vi "Init ConvBox Handler.vi"(8 "error in (no error)":errorcluster, 11 "Listener in":refnum<class "Listener.lvclass">) -> (0 "error out":errorcluster, 3 "Listener out":refnum<class "Listener.lvclass">)   [LabVIEW 2023, in "Listener.lvclass"]
uses:
  Listener.lvclass
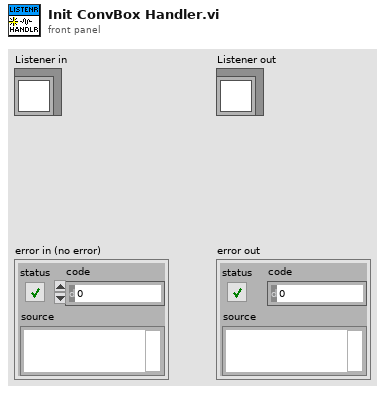
[diagram p1: front panel]
types:
  T1 = typedef "Listener.lvclass/RS-xxx To GPIB ConvBox Data Structure.ctl" = cluster{"Data":string, "Command Messages Read":string[], "Address":string, "Data Length":u32}
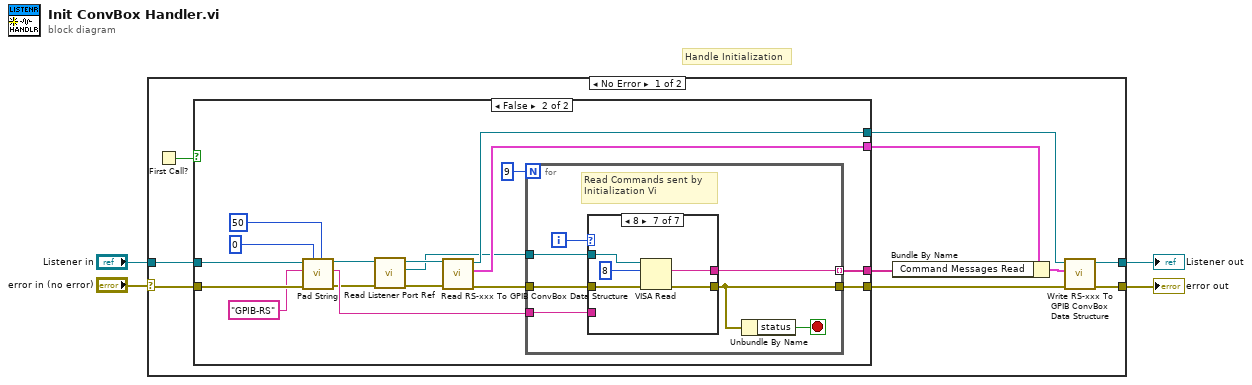
[diagram p0: block diagram]
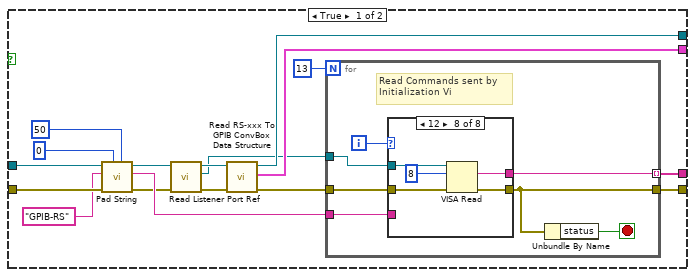
[diagram p2: hidden frame]
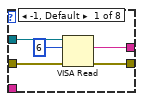
[diagram p3: hidden frame]
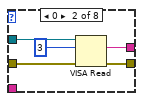
[diagram p4: hidden frame]
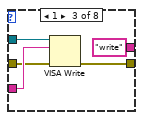
[diagram p5: hidden frame]
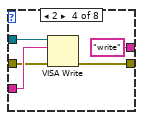
[diagram p6: hidden frame]
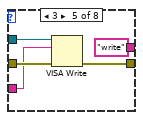
[diagram p7: hidden frame]
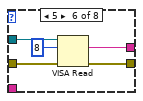
[diagram p8: hidden frame]
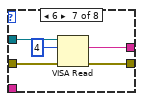
[diagram p9: hidden frame]
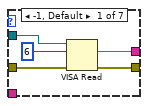
[diagram p10: hidden frame]
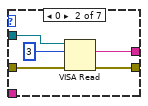
[diagram p11: hidden frame]
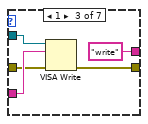
[diagram p12: hidden frame]
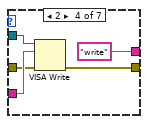
[diagram p13: hidden frame]
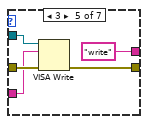
[diagram p14: hidden frame]
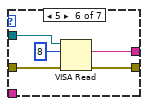
[diagram p15: hidden frame]
diagram:
  # "Handle Initialization"
  n1 = case shown="No Error" "error in (no error)" {
    selector: "error in (no error)" -> [w14 w139]
    tunnel: [w5 w139] -> w4
    tunnel: "Listener in" -> [w12 w138]
    tunnel: [w10 w138] -> w1
    frame No Error {
      n2 = First Call?() -> (First Call?: T/F=w13:bool)
      n3 = case shown="False" w13 {
        tunnel: [w31 w95] -> w6
        tunnel: w14 -> [w27 w91]
        tunnel: w12 -> [w22 w90]
        tunnel: [w29 w93] -> w11
        tunnel: [w21 w84] -> w9
        tunnel: [w20 w85] -> w8
        frame True {
          n4 = call "Pad String.vi"("Expected Length"=u8 50 ("Pad Character"), "Pad Character"=u8 0 ("Expected Length"), "error in (no error)"=w27, "String To Pad"="GPIB-RS" ("search string/char (-)"), "Listener in"=w22) -> ("error out"=w19:errorcluster, "Padded String"=w23:string, "Listener out"=w17:refnum<class "Listener.lvclass">)  [unwired: 4 in]
          n5 = call "Read Listener Port Ref.vi"("error in (no error)"=w19, "Listener in"=w17) -> ("error out"=w18:errorcluster, "Listener Port Ref"=w15:refnum<visa-resource-name>, "Listener out"=w16:refnum<class "Listener.lvclass">)  [unwired: 7 in]
          n6 = call-dynamic "Read RS-xxx To GPIB ConvBox Data Structure.vi"("error in (no error)"=w18, "Listener in"=w16) -> ("error out"=w28:errorcluster, "RS-xxx To GPIB ConvBox Data Structure"=w21:T1, "Listener out"=w29:refnum<class "Listener.lvclass">)  [unwired: 7 in]
          n7 = for {
            N: 13 -> [_]
            tunnel: w23 -> [w36]
            tunnel: [w34] -> w20 mode=indexing
            tunnel: w15 -> [w37]
            tunnel: w28 -> [w38]
            tunnel: [w33] -> w31
            i -> [w35]
            stop <- w32 stop-if-true
            # "Read Commands sent by\nInitialization Vi"
            n8 = case shown="12" w35 {
              tunnel: w38 -> [w43 w47 w51 w56 w62 w68 w73 w78]
              tunnel: w37 -> [w42 w48 w52 w57 w63 w67 w72 w77]
              tunnel: [w41 w45 w50 w55 w61 w66 w71 w76] -> w33
              tunnel: w36 -> [_ _ w53 w58 w59 _ _ _]
              tunnel: [w39 w44 "write" ("read buffer") "write" ("read buffer") "write" ("read buffer") w64 w69 w74] -> w34
              frame -1, Default {
                n9 = VISA Read(VISA resource name=w42, byte count=u32 6, error in (no error)=w43) -> (read buffer=w39:string, error out=w41:errorcluster)  [unwired: 2 out]
              }
              frame 0 {
                n10 = VISA Read(VISA resource name=w48, byte count=u32 3, error in (no error)=w47) -> (read buffer=w44:string, error out=w45:errorcluster)  [unwired: 2 out]
              }
              frame 1 {
                n11 = VISA Write(VISA resource name=w52, write buffer=w53, error in (no error)=w51) -> (error out=w50:errorcluster)  [unwired: 2 out]
              }
              frame 2 {
                n12 = VISA Write(VISA resource name=w57, write buffer=w58, error in (no error)=w56) -> (error out=w55:errorcluster)  [unwired: 2 out]
              }
              frame 3 {
                n13 = VISA Write(VISA resource name=w63, write buffer=w59, error in (no error)=w62) -> (error out=w61:errorcluster)  [unwired: 2 out]
              }
              frame 5 {
                n14 = VISA Read(VISA resource name=w67, byte count=u32 8, error in (no error)=w68) -> (read buffer=w64:string, error out=w66:errorcluster)  [unwired: 2 out]
              }
              frame 6 {
                n15 = VISA Read(VISA resource name=w72, byte count=u32 4, error in (no error)=w73) -> (read buffer=w69:string, error out=w71:errorcluster)  [unwired: 2 out]
              }
              frame 12 {
                n16 = VISA Read(VISA resource name=w77, byte count=u32 8, error in (no error)=w78) -> (read buffer=w74:string, error out=w76:errorcluster)  [unwired: 2 out]
              }
            }
            n17 = Unbundle By Name(w33) -> ("status"=w32:bool)
          }
        }
        frame False {
          n18 = call "Pad String.vi"("Expected Length"=u8 50, "Pad Character"=u8 0, "error in (no error)"=w91, "String To Pad"="GPIB-RS" ("search string/char (-)"), "Listener in"=w90) -> ("error out"=w80:errorcluster, "Padded String"=w86:string, "Listener out"=w81:refnum<class "Listener.lvclass">)  [unwired: 4 in]
          n19 = call "Read Listener Port Ref.vi"("error in (no error)"=w80, "Listener in"=w81) -> ("error out"=w83:errorcluster, "Listener Port Ref"=w79:refnum<visa-resource-name>, "Listener out"=w82:refnum<class "Listener.lvclass">)  [unwired: 7 in]
          n20 = call-dynamic "Read RS-xxx To GPIB ConvBox Data Structure.vi"("error in (no error)"=w83, "Listener in"=w82) -> ("error out"=w92:errorcluster, "RS-xxx To GPIB ConvBox Data Structure"=w84:T1, "Listener out"=w93:refnum<class "Listener.lvclass">)  [unwired: 7 in]
          n21 = for {
            N: 9 -> [_]
            tunnel: w79 -> [w101]
            tunnel: w86 -> [w100]
            tunnel: [w98] -> w85 mode=indexing
            tunnel: w92 -> [w102]
            tunnel: [w97] -> w95
            i -> [w99]
            stop <- w96 stop-if-true
            # "Read Commands sent by\nInitialization Vi"
            n22 = case shown="8" w99 {
              tunnel: w102 -> [w107 w111 w115 w120 w126 w132 w137]
              tunnel: w101 -> [w106 w112 w116 w121 w127 w131 w136]
              tunnel: [w105 w109 w114 w119 w125 w130 w135] -> w97
              tunnel: w100 -> [_ _ w117 w122 w123 _ _]
              tunnel: [w103 w108 "write" ("read buffer") "write" ("read buffer") "write" ("read buffer") w128 w133] -> w98
              frame -1, Default {
                n23 = VISA Read(VISA resource name=w106, byte count=u32 6, error in (no error)=w107) -> (read buffer=w103:string, error out=w105:errorcluster)  [unwired: 2 out]
              }
              frame 0 {
                n24 = VISA Read(VISA resource name=w112, byte count=u32 3, error in (no error)=w111) -> (read buffer=w108:string, error out=w109:errorcluster)  [unwired: 2 out]
              }
              frame 1 {
                n25 = VISA Write(VISA resource name=w116, write buffer=w117, error in (no error)=w115) -> (error out=w114:errorcluster)  [unwired: 2 out]
              }
              frame 2 {
                n26 = VISA Write(VISA resource name=w121, write buffer=w122, error in (no error)=w120) -> (error out=w119:errorcluster)  [unwired: 2 out]
              }
              frame 3 {
                n27 = VISA Write(VISA resource name=w127, write buffer=w123, error in (no error)=w126) -> (error out=w125:errorcluster)  [unwired: 2 out]
              }
              frame 5 {
                n28 = VISA Read(VISA resource name=w131, byte count=u32 8, error in (no error)=w132) -> (read buffer=w128:string, error out=w130:errorcluster)  [unwired: 2 out]
              }
              frame 8 {
                n29 = VISA Read(VISA resource name=w136, byte count=u32 8, error in (no error)=w137) -> (read buffer=w133:string, error out=w135:errorcluster)  [unwired: 2 out]
              }
            }
            n30 = Unbundle By Name(w97) -> ("status"=w96:bool)
          }
        }
      }
      n31 = Bundle By Name(cluster=w9, "Command Messages Read"=w8) -> (w7:T1)
      n32 = call-dynamic "Write RS-xxx To GPIB ConvBox Data Structure.vi"("error in (no error)"=w6, "RS-xxx To GPIB ConvBox Data Structure"=w7, "Listener in"=w11) -> ("error out"=w5:errorcluster, "Listener out"=w10:refnum<class "Listener.lvclass">)  [unwired: 7 in]
    }
    frame Error {
    }
  }
  "error out" <- w4
  "Listener out" <- w1
